vi "Pneumatic_Control_Initialize.vi"(9 "Forward?":bool, 10 "SolenoidDevRef":T1, 11 "name (unnamed)":string) -> (2 "Sense Loop":T5, 3 "Control Loop":T3)   [LabVIEW 2016]
doc: "Help by FRC Team 836 - The RoboBees\n\nThis VI initializes the pneumatic control & sensor loops."
uses:
  <userlib>/836-Libraries/Pneumatics/Support_Code/Pneumatic_Sensor_Loop.ctl
  <userlib>/836-Libraries/Pneumatics/Support_Code/Pneumatics_Status.ctl
  <vilib>/Rock Robotics/WPI/Solenoid/WPI_SolenoidValue.ctl
  <userlib>/836-Libraries/Pneumatics/Support_Code/Solenoid_Control_Loop.ctl
  <userlib>/836-Libraries/Pneumatics/Support_Code/Pneumatics_Command.ctl
  <userlib>/836-Libraries/Pneumatics/Support_Code/Pneumatics_Position.ctl
  <vilib>/Rock Robotics/WPI/Solenoid/WPI_SolenoidDevRef.ctl
  <vilib>/Rock Robotics/WPI/Solenoid/WPI_SolenoidChannel.ctl
  <vilib>/Rock Robotics/WPI/Solenoid/WPI_SolenoidSetEnum.vi
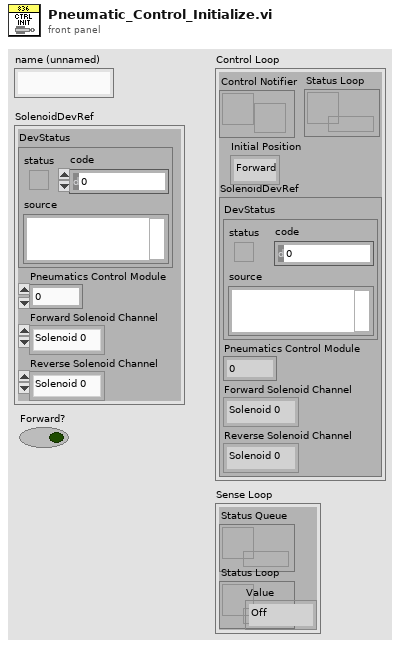
[diagram p1: front panel]
types:
  T1 = typedef "WPI_SolenoidDevRef.ctl" = cluster{"DevStatus":errorcluster, "Pneumatics Control Module":u8, "Forward Solenoid Channel":T2, "Reverse Solenoid Channel":T2}
  T2 = typedef "WPI_SolenoidChannel.ctl" = enum8{"Solenoid 0", "Solenoid 1", "Solenoid 2", "Solenoid 3", "Solenoid 4", "Solenoid 5", "Solenoid 6", "Solenoid 7", "Invalid"}
  T3 = typedef "Solenoid_Control_Loop.ctl" = cluster{"Control Notifier":refnum<notifier>, "Initial Position":T4, "SolenoidDevRef":T1, "Status Loop":refnum<k33>}
  T4 = typedef "Pneumatics_Position.ctl" = enum16{"Forward", "Reverse"}
  T5 = typedef "Pneumatic_Sensor_Loop.ctl" = cluster{"Status Queue":refnum<queue>, "Status Loop":refnum<k33>, "Relay Value":T6}
  T6 = typedef "WPI_SolenoidValue.ctl" = enum16{"Off", "On", "Forward", "Reverse"}
  T7 = typedef "Pneumatics_Command.ctl" = enum16{"Nothing", "Forward", "Reverse", "Toggle"}
  T8 = typedef "Pneumatics_Status.ctl" = enum16{"Forward", "Reverse", "Moving"}
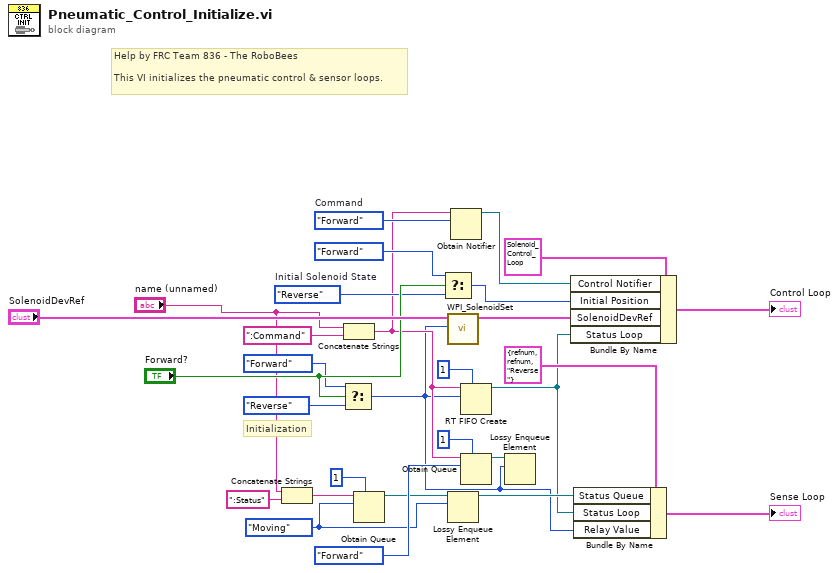
[diagram p0: block diagram]
diagram:
  w12 = Pneumatics_Command."Forward"  # Command
  w14 = Pneumatics_Status."Moving" ("Enum")
  w24 = Pneumatics_Position."Reverse"  # Initial Solenoid State
  # "Initialization"
  # "Help by FRC Team 836 - The RoboBees\n\nThis VI initializes the pneumatic control & sensor loops."
  n1 = Concatenate Strings("name (unnamed)", ":Status" ("string")) -> (w15:string)
  n2 = Select(t=WPI_SolenoidValue."Forward", s="Forward?", f=WPI_SolenoidValue."Reverse" ("Value")) -> (s? t:f=w1:T6)
  n3 = Concatenate Strings("name (unnamed)", ":Command" ("string")) -> (w4:string)
  n4 = Obtain Queue(max queue size (-1, unlimited)=1, name (unnamed)=w15, element data type=w14) -> (queue out=w6:refnum<queue>)  [unwired: 2 in, 2 out]
  n5 = Select(t=Pneumatics_Position."Forward", s="Forward?", f=w24) -> (s? t:f=w9:T4)
  n6 = call-poly <vilib>:"WPI_SolenoidSet.vi"("Value"=w1, "SolenoidDevRef"="SolenoidDevRef") -> ("SolenoidDevRef"=w8:T1)  [unwired: 8 in, 1 out]
  n7 = Lossy Enqueue Element(queue=w6, element=w14) -> (queue out=w5:refnum<queue>)  [unwired: 1 in, 3 out]
  n8 = Obtain Notifier(name (unnamed)=w4, notification data type=w12) -> (notifier out=w10:refnum<notifier>)  [unwired: 2 in, 2 out]
  n9 = RT FIFO Create(0:w4, 1:w1, 4:u32 1 ("size (10)")) -> (8:w3:refnum<k33>)  [unwired: 5 in, 2 out]
  n10 = Obtain Queue(max queue size (-1, unlimited)=1, name (unnamed)=w4, element data type=WPI_SolenoidValue."Forward" ("Value")) -> (queue out=w19:refnum<queue>)  [unwired: 2 in, 2 out]
  n11 = Lossy Enqueue Element(queue=w19, element=w1) -> ()  [unwired: 1 in, 4 out]
  n12 = Bundle By Name(cluster=T3 {"Control Notifier"=refnum, "Initial Position"=enum."Forward", "SolenoidDevRef"={"DevStatus"={"status"=FALSE, "code"=0, "source"=""}, "Pneumatics Control Module"=0, "Forward Solenoid Channel"=enum."Invalid", "Reverse Solenoid Channel"=enum."Invalid"}, "Status Loop"=refnum}, "Control Notifier"=w10, "Initial Position"=w9, "SolenoidDevRef"=w8, "Status Loop"=w3) -> (→"Control Loop":T3)
  n13 = Bundle By Name(cluster=T5 {"Status Queue"=refnum, "Status Loop"=refnum, "Relay Value"=enum."Reverse"}, "Status Queue"=w5, "Status Loop"=w3, "Relay Value"=w1) -> (→"Sense Loop":T5)
